vi "create incident - message.vi"(9 "message":string, 11 "RT Queues":T1) -> (3 "RT Queues out":T1)   [LabVIEW 2018]
uses:
  Type Defs/Queues cluster.ctl
  ICL-LabVIEW_General/Message Scheduler/message scheduler.lvclass
  Type Defs/generic incident.ctl
  Queue VIs/En-queue RT comms element.vi
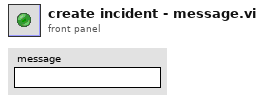
[diagram p1: front panel]
types:
  T1 = typedef "Queues cluster.ctl" = cluster{"RT Message":refnum<queue>, "RT Comms":refnum<queue>, "RT Data":refnum<queue>, "RT FIFO":refnum<queue>, "message scheduler":refnum<class "message scheduler.lvclass">}
  T2 = typedef "generic incident.ctl" = cluster{"timestamp":timestamp, "type":string, "Variant":variant}
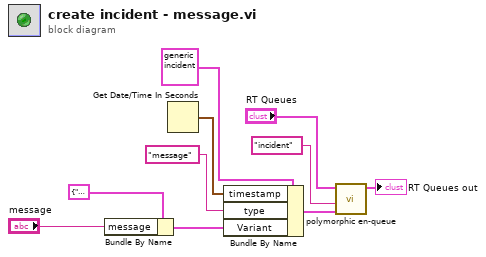
[diagram p0: block diagram]
diagram:
  n1 = Bundle By Name(cluster=cluster{"message":string, "data":variant} {"message"="", "data"=variant}, "message"="message") -> (w9:cluster{"message":string, "data":variant})
  n2 = Get Date/Time In Seconds() -> (seconds since 1Jan1904=w6:timestamp)
  n3 = Bundle By Name(cluster=T2 {"timestamp"=timestamp(0 s since 1904-01-01), "type"="", "Variant"=variant} ("incident cluster"), "timestamp"=w6, "type"="message", "Variant"=w9) -> (w5:T2)
  n4 = call-poly "polymorphic en-queue.vi"("Data"=w5, "Message"="incident", "RT Queues"="RT Queues") -> ("RT Queues out"=→"RT Queues out":T1)  [unwired: 8 in]
